vi "Util_Trajectory_WriteFile.vi"(4 "Trajectory is Cubic":bool, 5 "UseWeights":bool, 6 "Trajectory Is Relative":bool, 7 "TRAJECTORY_CONFIG":T1={"MaxVelocity"=0.0, "Max Acceleration"=0.0, "StartVelocity"=0.0, "End Velocity"=0.0, "Reversed"=FALSE, "DiffDrKineConstntDefined"=FALSE, "CentAcellConstntDefined"=FALSE, "DiffDrVoltConstntDefined"=FALSE, "DIFF_DRIVE_KINE_CONSTRAINT"={"Max Speed (M/S)"=0.0, "DIFF_DRIVE_KINEMATICS"={"TrackWidth_Meters"=0.0}}, "CENTRIPETAL_ACCEL_CONSTRAINT"={"Max Cent Accel"=0.0}, "SwerveDrKineConstntDefined"=FALSE, "SWERVE_DRIVE_KINE_CONSTRAINT"={"Max Speed (M/S)"=0.0, "SwerveKinematics"={"NumModules"=0, "InverseKinematics"=[], "ForwardKinematics"=[], "Modules"=[], "PrevCoR"={"X"=0.0, "Y"=0.0}}}, "DIFF_DRIVE_VOLTAGE_CONSTRAINT"={"Max Voltage"=0.0, "DIFF_DRIVE_KINEMATICS"={"TrackWidth_Meters"=0.0}, "SIMPLE_MOTOR_FF"={"Ks"=0.0, "Kv"=0.0, "Ka"=0.0}}, "MECANUM_DRIVE_KINE_CONSTRAINT"={"Max Speed (M/S)"=0.0, "MECA_DRIVE_KINEMATICS"={"FrontLeft"={"X"=0.0, "Y"=0.0}, "FrontRight"={"X"=0.0, "Y"=0.0}, "RearLeft"={"X"=0.0, "Y"=0.0}, "RearRight"={"X"=0.0, "Y"=0.0}, "InverseKinematics"=[[0.0, 1.0, -1.0, 0.0], [0.0, 1.0, 1.0, 0.0], [0.0, 1.0, 1.0, 0.0], [0.0, 1.0, -1.0, 0.0]], "ForwardKinematics"=[[0.0, 1.0, -1.0, 0.0], [0.0, 1.0, 1.0, 0.0], [0.0, 1.0, 1.0, 0.0], [0.0, 1.0, -1.0, 0.0]], "PrevCoR"={"X"=0.0, "Y"=0.0}}}, "MecanumDrKineConstntDefined"=FALSE} {"MECANUM_DRIVE_KINE_CONSTRAINT"."MECA_DRIVE_KINEMATICS"."PrevCoR"."Y" format="%14.3f"; "MECANUM_DRIVE_KINE_CONSTRAINT"."MECA_DRIVE_KINEMATICS"."PrevCoR"."X" format="%14.3f"; "MECANUM_DRIVE_KINE_CONSTRAINT"."MECA_DRIVE_KINEMATICS"."RearRight"."Y" format="%14.3f"; "MECANUM_DRIVE_KINE_CONSTRAINT"."MECA_DRIVE_KINEMATICS"."RearRight"."X" format="%14.3f"; "MECANUM_DRIVE_KINE_CONSTRAINT"."MECA_DRIVE_KINEMATICS"."RearLeft"."Y" format="%14.3f"; "MECANUM_DRIVE_KINE_CONSTRAINT"."MECA_DRIVE_KINEMATICS"."RearLeft"."X" format="%14.3f"; "MECANUM_DRIVE_KINE_CONSTRAINT"."MECA_DRIVE_KINEMATICS"."FrontRight"."Y" format="%14.3f"; "MECANUM_DRIVE_KINE_CONSTRAINT"."MECA_DRIVE_KINEMATICS"."FrontRight"."X" format="%14.3f"; "MECANUM_DRIVE_KINE_CONSTRAINT"."MECA_DRIVE_KINEMATICS"."FrontLeft"."Y" format="%14.3f"; "MECANUM_DRIVE_KINE_CONSTRAINT"."MECA_DRIVE_KINEMATICS"."FrontLeft"."X" format="%14.3f"; "MECANUM_DRIVE_KINE_CONSTRAINT"."Max Speed (M/S)" format="%20.4f"; "DIFF_DRIVE_VOLTAGE_CONSTRAINT"."SIMPLE_MOTOR_FF"."Ka" format="%13.4f"; "DIFF_DRIVE_VOLTAGE_CONSTRAINT"."SIMPLE_MOTOR_FF"."Kv" format="%13.4f"; "DIFF_DRIVE_VOLTAGE_CONSTRAINT"."SIMPLE_MOTOR_FF"."Ks" format="%13.4f"; "DIFF_DRIVE_VOLTAGE_CONSTRAINT"."DIFF_DRIVE_KINEMATICS"."TrackWidth_Meters" format="%20.4f"; "DIFF_DRIVE_VOLTAGE_CONSTRAINT"."Max Voltage" format="%20.4f"; "SWERVE_DRIVE_KINE_CONSTRAINT"."SwerveKinematics"."PrevCoR"."Y" format="%14.3f"; "SWERVE_DRIVE_KINE_CONSTRAINT"."SwerveKinematics"."PrevCoR"."X" format="%14.3f"; "SWERVE_DRIVE_KINE_CONSTRAINT"."SwerveKinematics"."Modules"."Y" format="%14.3f"; "SWERVE_DRIVE_KINE_CONSTRAINT"."SwerveKinematics"."Modules"."X" format="%14.3f"; "SWERVE_DRIVE_KINE_CONSTRAINT"."Max Speed (M/S)" format="%20.4f"; "CENTRIPETAL_ACCEL_CONSTRAINT"."Max Cent Accel" format="%20.4f"; "DIFF_DRIVE_KINE_CONSTRAINT"."DIFF_DRIVE_KINEMATICS"."TrackWidth_Meters" format="%20.4f"; "DIFF_DRIVE_KINE_CONSTRAINT"."Max Speed (M/S)" format="%20.4f"; "End Velocity" format="%20.4f"; "StartVelocity" format="%20.4f"; "Max Acceleration" format="%20.4f"; "MaxVelocity" format="%20.4f"}, 8 "UtilityWayPoints":T13[](array[typedef]) {"WEIGHT" format="%13.3f"; "ANGLE" format="%13.3f"; "Y" format="%13.3f"; "X" format="%13.3f"}, 9 "TRAJECTORY":T14 {"States"."POSE"."ROTATION"."SIN" format="%13.4f"; "States"."POSE"."ROTATION"."COS" format="%13.4f"; "States"."POSE"."ROTATION"."VALUE" format="%13.4f"; "States"."POSE"."TRANSLATION"."Y" format="%14.3f"; "States"."POSE"."TRANSLATION"."X" format="%14.3f"; "TotalTImeSecs" format="%20.3f"}, 10 "Comment":string, 11 "Trajectory File Name":path) -> (0 "error out":errorcluster)   [LabVIEW 2019, in "Trajectory_Library.lvlib"]
doc: "Create a CSV file from a Trajectory data structure. This can be used on a PC or the RoboRIO.\n\nParameters:\n - Trajectory - Data structure containing trajectory\n - TrajectoryConfig - Trajectory configuration\n - Trajectory File Name - File name to write to. Existing files are overwritten.\n - Comment - Comment string to include in file comments.\n - Waypoints - waypoints to include in file comments\n - TrajectoryIsRelative - Relative if TRUE otherwise absolute\n - TrajectoryIsCubic - Cubic if TRUE otherwise Quintic\n\nReturns:\n - Error out - returned error cluster\n\nReturns:\n - outTrajectory - Trajectory data structure\n - Error out - returned error cluster"
uses:
  Trajectory_Library.lvlib
  TRAJECTORY.ctl
  TRAJ_STATE.ctl
  POSE2D.ctl
  TRANSLATION2D.ctl
  ROTATION2D.ctl
  UTIL_WEIGHTED_WAYPOINT.ctl
  TRAJ_CONFIG.ctl
  TRAJ_CONSTRAINT_DIIF_DRIVE_KINEMATICS.ctl
  DIFF_DRIVE_KINEMATICS.ctl
  TRAJ_CONSTRAINT_CENTRIPETAL_ACCEL.ctl
  TRAJ_CONSTRAINT_SWERVE_DRIVE_KINEMATICS.ctl
  SWERVE_DRIVE_KINEMATICS.ctl
  <vilib>/Analysis/Matrix/Datatypes/RealMatrix.ctl
  TRAJ_CONSTRAINT_DIIF_DRIVE_VOLTAGE.ctl
  SIMPLE_MOTOR_FF.ctl
  TRAJ_CONSTRAINT_MECA_DRIVE_KINEMATICS.ctl
  MECA_DRIVE_KINEMATICS.ctl
  <vilib>/Analysis/Matrix/NI_Matrix.lvlib
panel:
  # "ARRAY OF OTHER\nCONSTRAINTS \nGOES HERE.."
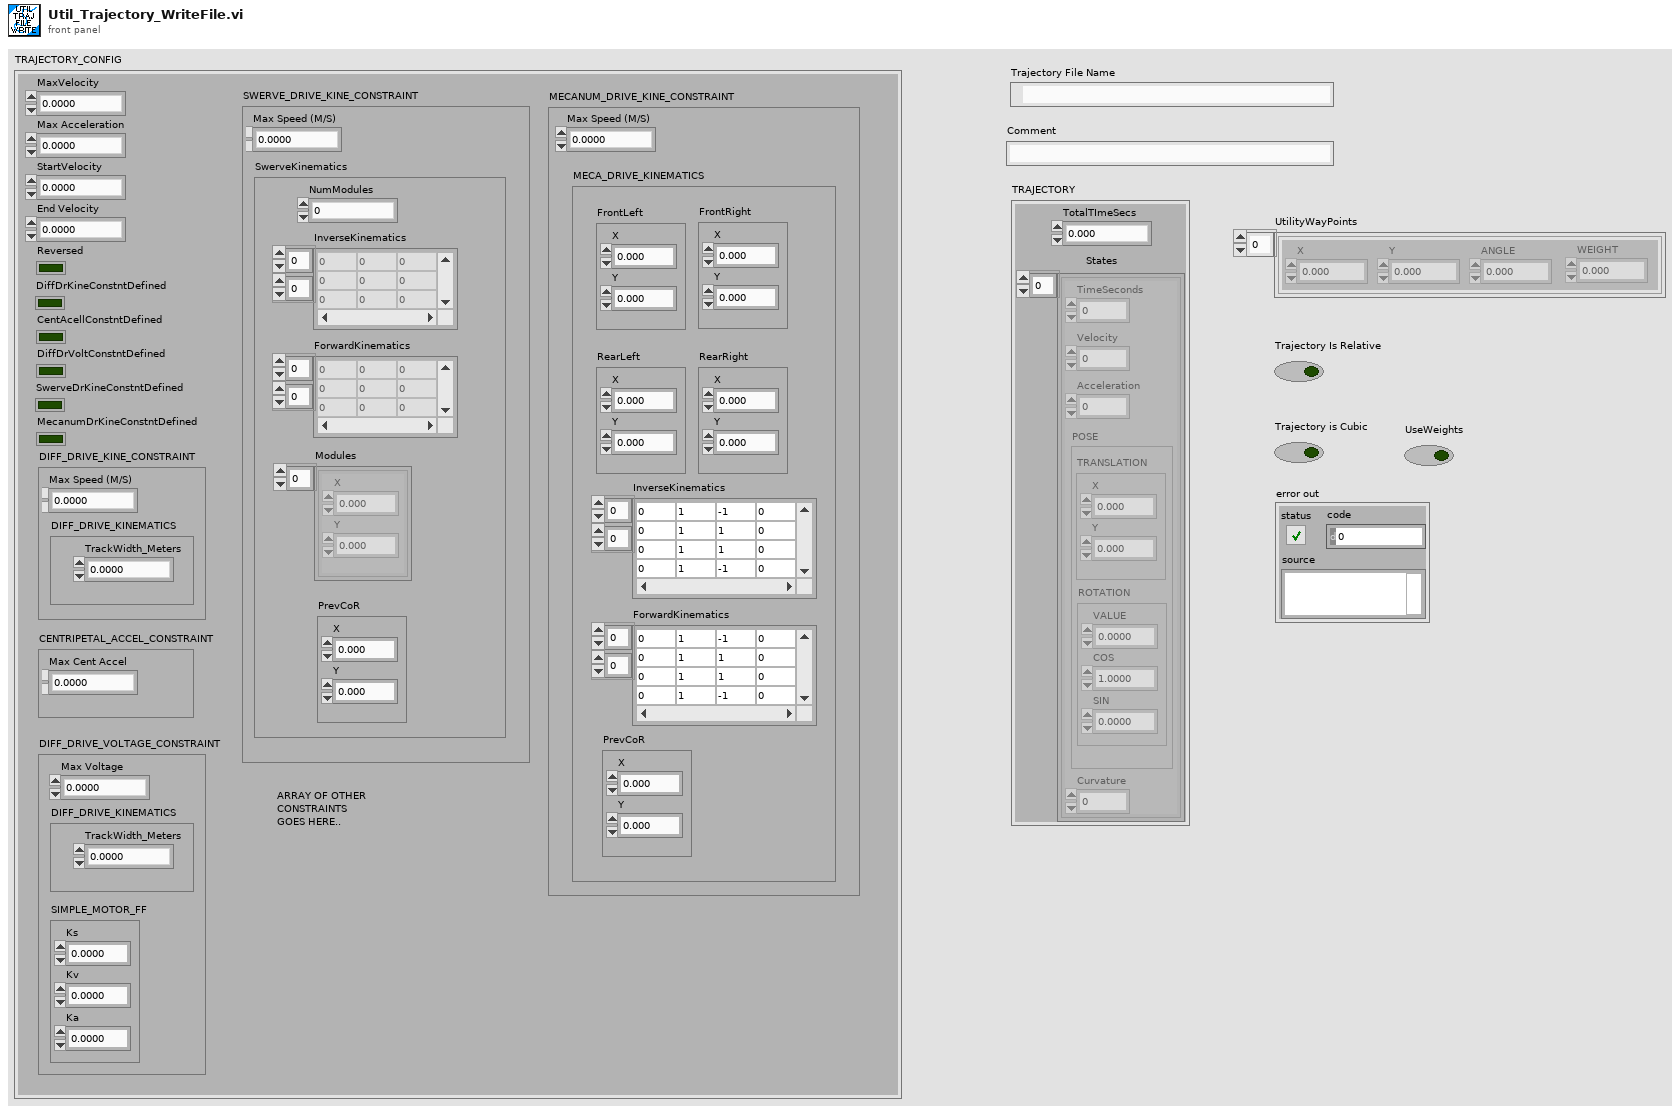
[diagram p1: front panel]
types:
  T1 = typedef "Trajectory_Library.lvlib/TRAJ_CONFIG.ctl" = cluster{"MaxVelocity":dbl, "Max Acceleration":dbl, "StartVelocity":dbl, "End Velocity":dbl, "Reversed":bool, "DiffDrKineConstntDefined":bool, "CentAcellConstntDefined":bool, "DiffDrVoltConstntDefined":bool, "DIFF_DRIVE_KINE_CONSTRAINT":T2, "CENTRIPETAL_ACCEL_CONSTRAINT":T4, "SwerveDrKineConstntDefined":bool, "SWERVE_DRIVE_KINE_CONSTRAINT":T5, "DIFF_DRIVE_VOLTAGE_CONSTRAINT":T9, "MECANUM_DRIVE_KINE_CONSTRAINT":T11, "MecanumDrKineConstntDefined":bool}
  T2 = typedef "Trajectory_Library.lvlib/TRAJ_CONSTRAINT_DIIF_DRIVE_KINEMATICS.ctl" = cluster{"Max Speed (M/S)":dbl, "DIFF_DRIVE_KINEMATICS":T3}
  T3 = typedef "Trajectory_Library.lvlib/DIFF_DRIVE_KINEMATICS.ctl" = cluster{"TrackWidth_Meters":dbl}
  T4 = typedef "Trajectory_Library.lvlib/TRAJ_CONSTRAINT_CENTRIPETAL_ACCEL.ctl" = cluster{"Max Cent Accel":dbl}
  T5 = typedef "Trajectory_Library.lvlib/TRAJ_CONSTRAINT_SWERVE_DRIVE_KINEMATICS.ctl" = cluster{"Max Speed (M/S)":dbl, "SwerveKinematics":T6}
  T6 = typedef "Trajectory_Library.lvlib/SWERVE_DRIVE_KINEMATICS.ctl" = cluster{"NumModules":i32, "InverseKinematics":T7, "ForwardKinematics":T7, "Modules":T8[], "PrevCoR":T8}
  T7 = typedef "NI_Matrix.lvlib/RealMatrix.ctl" = dbl[][]
  T8 = typedef "Trajectory_Library.lvlib/TRANSLATION2D.ctl" = cluster{"X":dbl, "Y":dbl}
  T9 = typedef "Trajectory_Library.lvlib/TRAJ_CONSTRAINT_DIIF_DRIVE_VOLTAGE.ctl" = cluster{"Max Voltage":dbl, "DIFF_DRIVE_KINEMATICS":T3, "SIMPLE_MOTOR_FF":T10}
  T10 = typedef "Trajectory_Library.lvlib/SIMPLE_MOTOR_FF.ctl" = cluster{"Ks":dbl, "Kv":dbl, "Ka":dbl}
  T11 = typedef "Trajectory_Library.lvlib/TRAJ_CONSTRAINT_MECA_DRIVE_KINEMATICS.ctl" = cluster{"Max Speed (M/S)":dbl, "MECA_DRIVE_KINEMATICS":T12}
  T12 = typedef "Trajectory_Library.lvlib/MECA_DRIVE_KINEMATICS.ctl" = cluster{"FrontLeft":T8, "FrontRight":T8, "RearLeft":T8, "RearRight":T8, "InverseKinematics":T7, "ForwardKinematics":T7, "PrevCoR":T8}
  T13 = typedef "Trajectory_Library.lvlib/UTIL_WEIGHTED_WAYPOINT.ctl" = cluster{"X":dbl, "Y":dbl, "ANGLE":dbl, "WEIGHT":dbl}
  T14 = typedef "Trajectory_Library.lvlib/TRAJECTORY.ctl" = cluster{"TotalTImeSecs":dbl, "States":T15[]}
  T15 = typedef "Trajectory_Library.lvlib/TRAJ_STATE.ctl" = cluster{"TimeSeconds":dbl, "Velocity":dbl, "Acceleration":dbl, "POSE":T16, "Curvature":dbl}
  T16 = typedef "Trajectory_Library.lvlib/POSE2D.ctl" = cluster{"TRANSLATION":T8, "ROTATION":T17}
  T17 = typedef "Trajectory_Library.lvlib/ROTATION2D.ctl" = cluster{"VALUE":dbl, "COS":dbl, "SIN":dbl}
  T18 = enum16{"open", "replace", "create", "open or create", "replace or create", "replace or create with confirmation"}
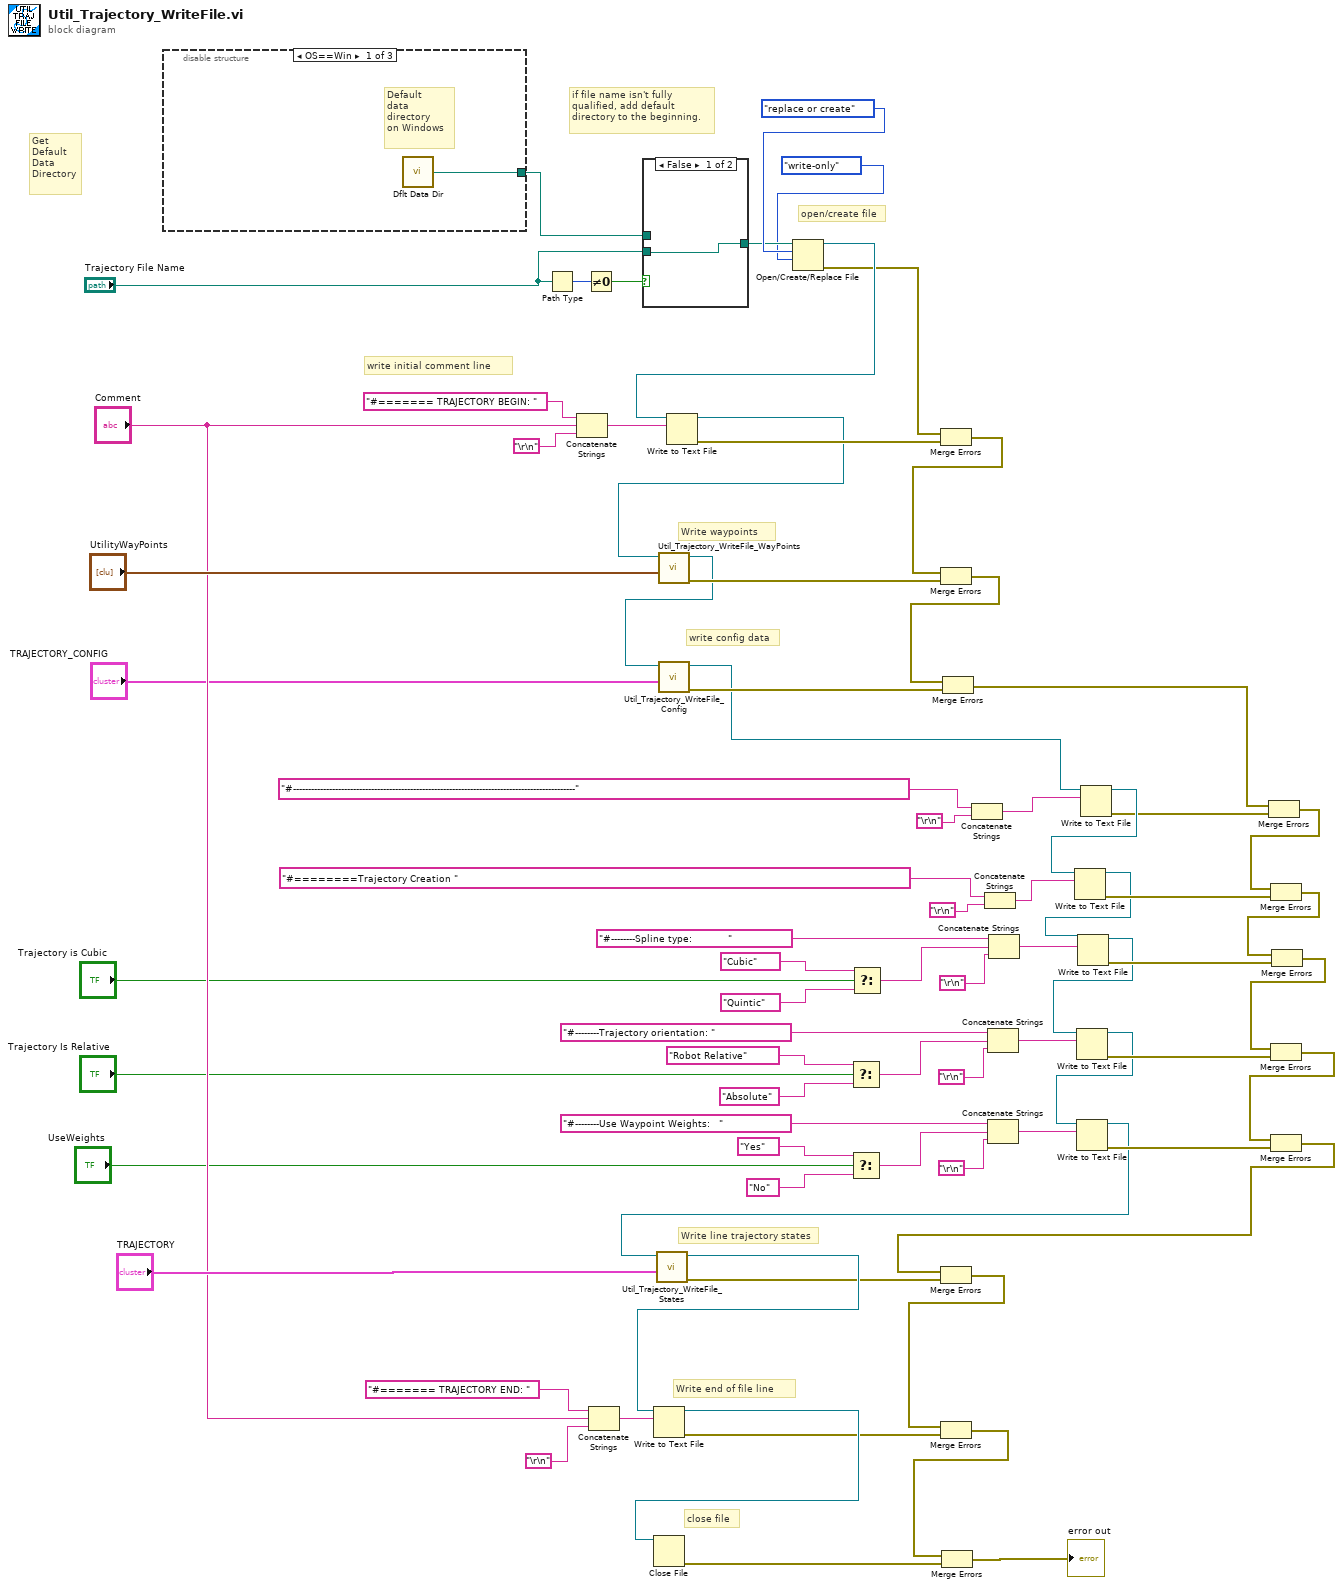
[diagram p0: block diagram]
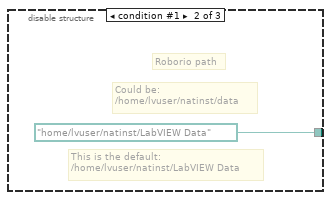
[diagram p2: hidden frame]
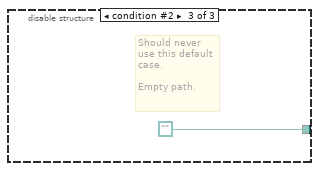
[diagram p3: hidden frame]
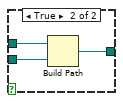
[diagram p4: hidden frame]
diagram:
  # "write config data"
  # "Write line trajectory states"
  # "open/create file"
  # "if file name isn't fully \nqualified, add default\ndirectory to the beginning."
  # "Get\nDefault\nData\nDirectory"
  # "Write waypoints"
  # "close file"
  # "Write end of file line"
  # "write initial comment line"
  n1 = disable-structure shown="OS==Win" {
    disable-tunnel: [w79 path "/home/lvuser/natinst/LabVIEW Data" path ""] -> w68
    frame condition #0 (active) {
      # "Default\ndata\ndirectory\non Windows"
      n2 = call <vilib>:"Dflt Data Dir.vi"() -> ("App:Default Data Directory"=w79:path)
    }
    frame condition #1 {
      # "This is the default:\n/home/lvuser/natinst/LabVIEW Data"
      # "Could be:\n/home/lvuser/natinst/data"
      # "Roborio path"
    }
    frame condition #2 {
      # "Should never\nuse this default\ncase.\n\nEmpty path."
    }
  }
  n3 = Path Type(1:"Trajectory File Name") -> (0:w71:i16)
  n4 = Concatenate Strings("#======= TRAJECTORY BEGIN: " ("string"), "Comment", "\r\n") -> (w76:string)
  n5 = Not Equal To 0?(x=w71) -> (x != 0?=w70:bool)
  n6 = Concatenate Strings("#======= TRAJECTORY END: " ("string"), "Comment", "\r\n") -> (w72:string)
  n7 = case shown="False" w70 {
    tunnel: [w82 w85] -> w67
    tunnel: w68 -> [_ w84]
    tunnel: "Trajectory File Name" -> [w82 w83]
    frame False {
    }
    frame True {
      n8 = Build Path(base path=w84, name or relative path=w83) -> (appended path=w85:path)
    }
  }
  n9 = Open/Create/Replace File(file path (use dialog)=w67, operation (0:open)=T18."replace or create", access (0:read/write)=enum16{"read/write", "read-only", "write-only"}."write-only") -> (refnum out=w63:refnum<file>, error out=w58:errorcluster)  [unwired: 3 in, 1 out]
  n10 = Write to Text File(file (use dialog)=w63, text=w76) -> (refnum out=w49:refnum<file>, error out=w59:errorcluster)  [unwired: 2 in, 1 out]
  n11 = call "Util_Trajectory_WriteFile_WayPoints.vi"("UtilityWayPoints"="UtilityWayPoints", "Byte Steam File In"=w49) -> ("error out"=w57:errorcluster, "Byte Steam File Out"=w47:refnum<file>)  [unwired: 8 in]
  n12 = call "Util_Trajectory_WriteFile_Config.vi"("TRAJECTORY_CONFIG"="TRAJECTORY_CONFIG", "Byte Steam File In"=w47) -> ("error out"=w46:errorcluster, "Byte Steam File Out"=w27:refnum<file>)  [unwired: 8 in]
  n13 = Select(t="Robot Relative" ("string"), s="Trajectory Is Relative", f="Absolute" ("string")) -> (s? t:f=w35:string)
  n14 = Select(t="Yes" ("string"), s="UseWeights", f="No" ("string")) -> (s? t:f=w9:string)
  n15 = Select(t="Cubic" ("string"), s="Trajectory is Cubic", f="Quintic" ("string")) -> (s? t:f=w21:string)
  n16 = Merge Errors(w58, w59) -> (w50:errorcluster)
  n17 = Merge Errors(w50, w57) -> (w45:errorcluster)
  n18 = Merge Errors(w45, w46) -> (w25:errorcluster)
  n19 = Concatenate Strings("#----------------------------------------------------------------------------------------------" ("string"), "\r\n") -> (w39:string)
  n20 = Concatenate Strings("#========Trajectory Creation " ("string"), "\r\n") -> (w42:string)
  n21 = Concatenate Strings("#--------Trajectory orientation: " ("string"), w35, "\r\n") -> (w37:string)
  n22 = Concatenate Strings("#--------Use Waypoint Weights:   " ("string"), w9, "\r\n") -> (w11:string)
  n23 = Concatenate Strings("#--------Spline type:            " ("string"), w21, "\r\n") -> (w23:string)
  n24 = Write to Text File(file (use dialog)=w27, text=w39) -> (refnum out=w31:refnum<file>, error out=w29:errorcluster)  [unwired: 2 in, 1 out]
  n25 = Write to Text File(file (use dialog)=w31, text=w42) -> (refnum out=w17:refnum<file>, error out=w30:errorcluster)  [unwired: 2 in, 1 out]
  n26 = Write to Text File(file (use dialog)=w17, text=w23) -> (refnum out=w16:refnum<file>, error out=w22:errorcluster)  [unwired: 2 in, 1 out]
  n27 = Write to Text File(file (use dialog)=w16, text=w37) -> (refnum out=w3:refnum<file>, error out=w36:errorcluster)  [unwired: 2 in, 1 out]
  n28 = Write to Text File(file (use dialog)=w3, text=w11) -> (refnum out=w2:refnum<file>, error out=w10:errorcluster)  [unwired: 2 in, 1 out]
  n29 = call "Util_Trajectory_WriteFile_States.vi"("Trajectory"="TRAJECTORY", "Byte Steam File In"=w2) -> ("error out"=w56:errorcluster, "Byte Steam File Out"=w61:refnum<file>)  [unwired: 8 in]
  n30 = Write to Text File(file (use dialog)=w61, text=w72) -> (refnum out=w60:refnum<file>, error out=w54:errorcluster)  [unwired: 2 in, 1 out]
  n31 = Close File(refnum=w60) -> (error out=w53:errorcluster)  [unwired: 1 in, 1 out]
  n32 = Merge Errors(w25, w29) -> (w28:errorcluster)
  n33 = Merge Errors(w28, w30) -> (w15:errorcluster)
  n34 = Merge Errors(w15, w22) -> (w14:errorcluster)
  n35 = Merge Errors(w14, w36) -> (w5:errorcluster)
  n36 = Merge Errors(w5, w10) -> (w4:errorcluster)
  n37 = Merge Errors(w4, w56) -> (w55:errorcluster)
  n38 = Merge Errors(w55, w54) -> (w52:errorcluster)
  n39 = Merge Errors(w52, w53) -> (→"error out":errorcluster)
